vi "String to Double (Division).vi"(1 "String":string) -> (0 "Number":dbl)   [LabVIEW 2013]
doc: "Parses a string to a number."
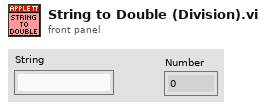
[diagram p1: front panel]
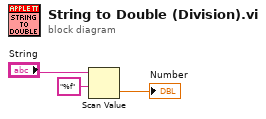
[diagram p0: block diagram]
diagram:
  n1 = Scan Value(string="String", format string="%f") -> (value=→"Number":dbl)  [unwired: 1 in, 1 out]
